vi "Read Timing Status.vi"(8 "error in (no error)":errorcluster, 11 "Framework Performance in":refnum<class "Performance.lvclass">) -> (0 "error out":errorcluster, 2 "timing status":T1 {"prev start time" format="%d us"; "cycle end time" format="%d us"; "cycle start time" format="%d us"; "tx end time" format="%d us"; "tx start time" format="%d us"; "rx end time" format="%d us"; "rx start time" format="%d us"}, 3 "Framework Performance out":refnum<class "Performance.lvclass">)   [LabVIEW 2017, in "DSF Core.lvlib" / "Performance.lvclass"]
uses:
  Performance.lvclass
  Timing Status/Timing Status Data.ctl
  Performance.lvclass/Performance.ctl
  Timing Status/Timing Status.lvclass
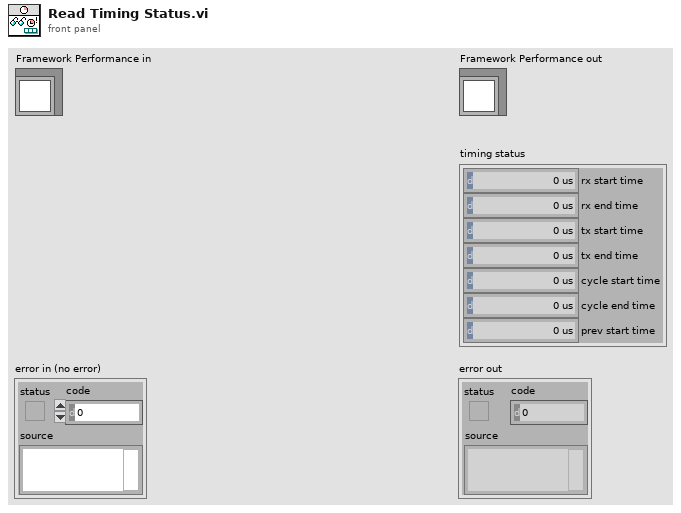
[diagram p1: front panel]
types:
  T1 = typedef "DSF Core.lvlib/Timing Status.lvclass/Timing Status Data.ctl" = cluster{"rx start time":u32, "rx end time":u32, "tx start time":u32, "tx end time":u32, "cycle start time":u32, "cycle end time":u32, "prev start time":u32}
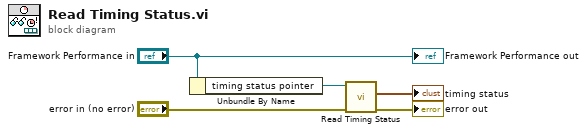
[diagram p0: block diagram]
diagram:
  n1 = Unbundle By Name("Framework Performance in") -> ("timing status pointer"=w4:refnum<class "Timing Status.lvclass">)
  n2 = call "Read Timing Status.vi"("error in (no error)"="error in (no error)", "timing status pointer in"=w4) -> ("error out"=→"error out":errorcluster, "timing status"=→"timing status":T1)  [unwired: 7 in, 1 out]
  "Framework Performance out" <- "Framework Performance in"
